vi "LOERN Tester.vi"() -> ()   [LabVIEW 2016]
uses:
  <vilib>/LIEF/Image Editor Handler/Image Editor Handler.lvclass
panel:
  out "class path":path
  out "class name":string
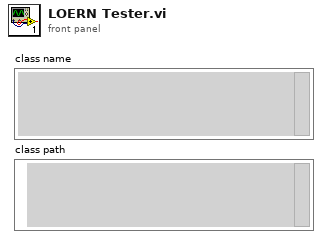
[diagram p1: front panel]
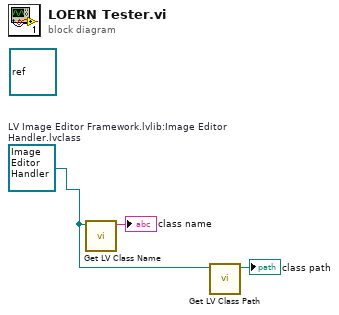
[diagram p0: block diagram]
diagram:
  w1 = refnum<class "Image Editor Handler.lvclass"> refnum  # LV Image Editor Framework.lvlib:Image Editor Handler.lvclass
  (unwired) refnum<class> refnum ("LabVIEW Object")
  n1 = call <vilib>:"Get LV Class Name.vi"("object"=w1) -> ("class name"=→"class name":string)  [unwired: 9 in, 1 out]
  n2 = call <vilib>:"Get LV Class Path.vi"("object"=w1) -> ("class path"=→"class path":path)  [unwired: 9 in, 1 out]
